vi "LoadRecalcSave.vi"(6 "Segments":bool[](array[boolean]), 8 "Time":string, 9 "Segments(s)":dbl[](array[numeric]), 10 "LoadBackPath":path, 11 "Slide in":refnum<vi>) -> (2 "ForAnalysisPath":path, 3 "ForSegmentsBMP":path)   [LabVIEW 2018]
uses:
  <vilib>/Utility/file.llb/Write Delimited Spreadsheet (string).vi
  Globaltracker.vi
panel:
  out "TTLIsActive":bool
  out "TTLOn":i32
  out "Counter":i32
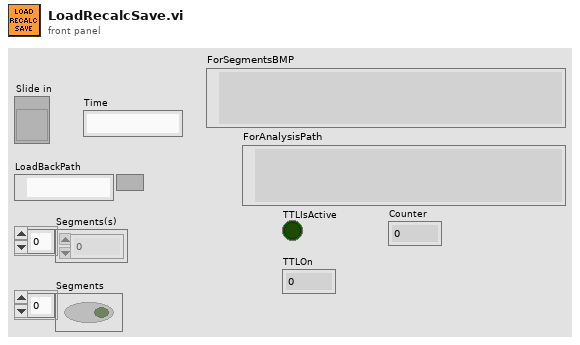
[diagram p1: front panel]
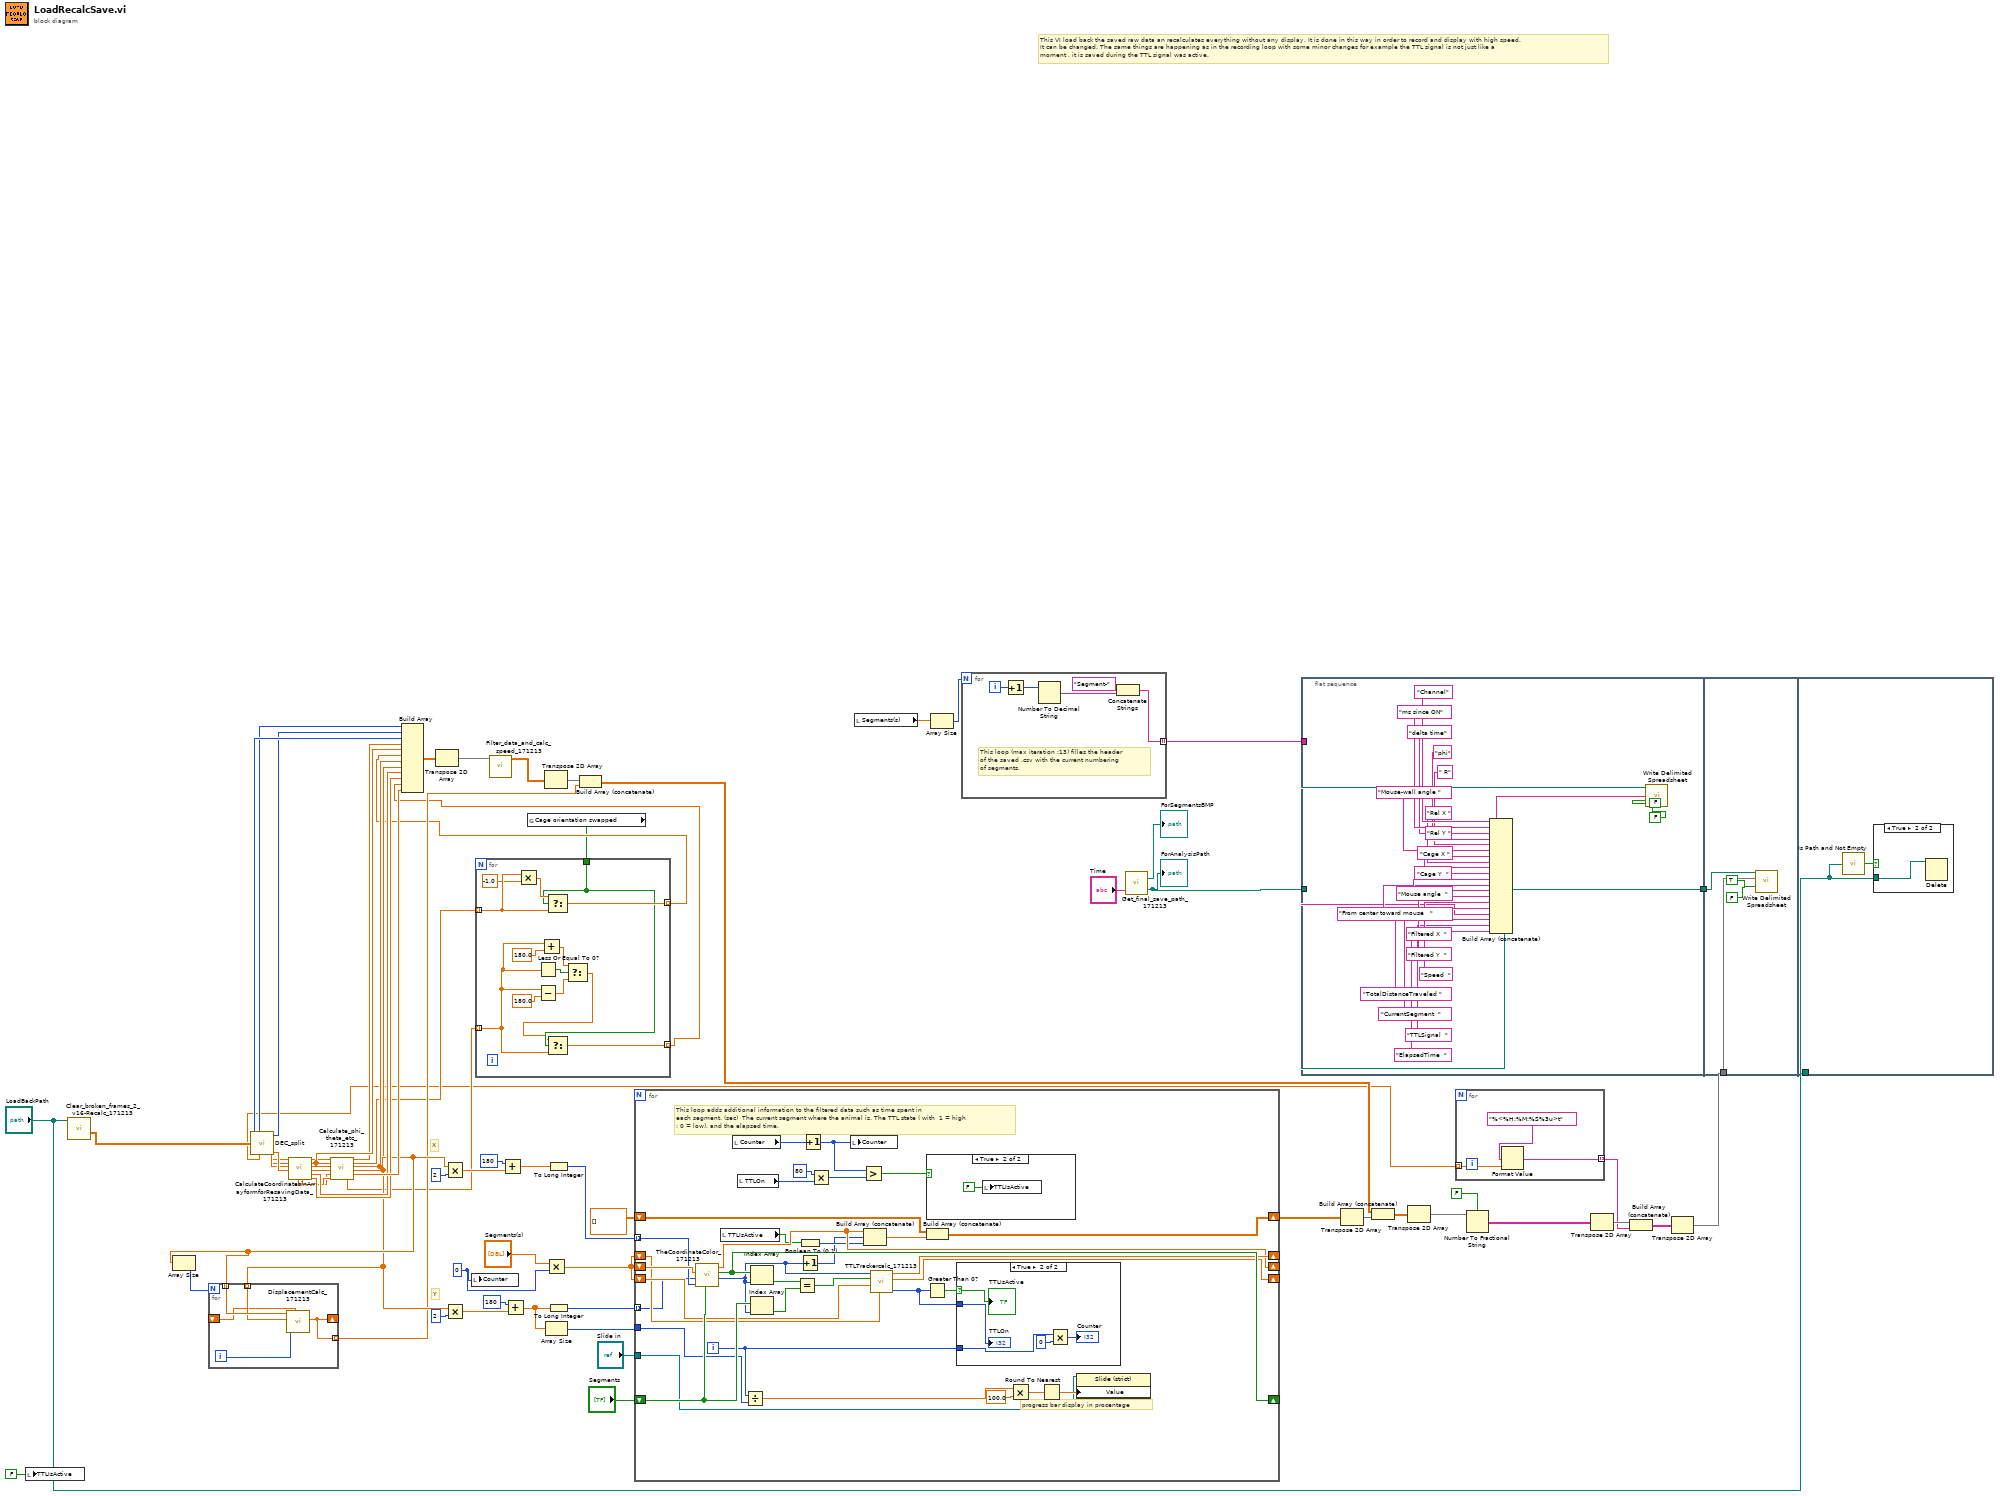
[diagram p0: block diagram]
diagram:
  w23 = 0 ("index")
  # "This VI load back the saved raw data an recalculates everything without any display. It is done in this way in order to record and display with high speed. \nIt can be changed. The same things are happening as in the recording loop with some minor changes for example the TTL signal is not just like a\nmoment , it is saved during the TTL signal was active."
  # "Y"
  # "X"
  n1 = local write "TTLIsActive"(FALSE ("TTLIsActive")) -> ()
  n2 = call "Clear_broken_frames_2_v16-Recalc_171213.vi"("file path (dialog if empty)"="LoadBackPath") -> ("Cleaned array"=w16:dbl[][])  [unwired: 8 in, 2 out]
  n3 = call "DEC_split.vi"("Input DEC array"=w16) -> ("ms since ON"=w39:u32[], "Channel"=w38:u32[], "delta time"=w40:u32[], "Timepoint"=w1:dbl[], "X1"=w29:sgl[], "Y1"=w30:sgl[], "X2"=w31:sgl[], "Y2"=w32:sgl[])  [unwired: 2 out]
  n4 = call "CalculateCoordinatesinArrayformforResavingData_171213.vi"("X1"=w29, "Y1"=w30, "X2"=w31, "Y2"=w32) -> ("X1-X2"=w36:sgl[], "Y1-Y2"=w37:sgl[], "sin(a)"=w33:sgl[], "R from center"=w42:sgl[], "Mouse Xc"=w34:sgl[], "Mouse Yc"=w35:sgl[], "Cage Xc"=w43:sgl[], "Cage Yc"=w44:sgl[])  [unwired: 8 in]
  n5 = call "Calculate_phi_theta_etc_171213.vi"("sin(a)"=w33, "R from center"=w42, "Mouse Xc"=w34, "Mouse Yc"=w35, "X1-X2"=w36, "Y1-Y2"=w37) -> ("Mouse-angle"=w7:dbl[], "phi"=w41:dbl[], "Mouse-wall angle"=w6:dbl[], "Rel X"=w13:dbl[], "Rel Y"=w12:dbl[], "From center towards mouse"=w45:dbl[])  [unwired: 7 in, 1 out]
  n6 = Array Size(array=w13) -> (size(s)=w14:i32)
  n7 = for {
    N: w14 -> [_]
    tunnel: w13 -> [w73] mode=indexing
    tunnel: w12 -> [w72] mode=indexing
    shift-right: [w70] -> _
    shift-left: _ -> [w71]
    tunnel: [w70] -> w9 mode=indexing
    i -> [w74]
    n8 = call "DisplacementCalc_171213.vi"("TotalDistanceTraveledInput"=w71, "i"=w74, "Y"=w72, "X"=w73) -> ("TotalDistanceTraveledOutput"=w70:dbl)  [unwired: 6 in, 1 out]
  }
  n9 = Multiply(x=w13, y=2 ("disabled index (col)")) -> (x*y=w49:dbl[])
  n10 = Multiply(x=w12, y=2 ("disabled index (col)")) -> (x*y=w50:dbl[])
  n11 = local write "Counter"(w23) -> ()
  n12 = Add(x=180 ("disabled index (col)"), y=w49) -> (x+y=w53:dbl[])
  n13 = Add(x=180 ("disabled index (col)"), y=w50) -> (x+y=w68:dbl[])
  n14 = global read "Globaltracker.vi" "Cage orientation swapped"() -> (w4:bool)
  n15 = for {
    tunnel: w7 -> [w76] mode=indexing
    tunnel: w6 -> [w85] mode=indexing
    tunnel: [w87] -> w5 mode=indexing
    tunnel: w4 -> [w82]
    tunnel: [w83] -> w3 mode=indexing
    n16 = Multiply(x=w85, y=-1.0) -> (x*y=w86:dbl)
    n17 = Less Or Equal To 0?(x=w76) -> (x <= 0?=w81:bool)
    n18 = Subtract(x=w76, y=180.0) -> (x-y=w77:dbl)
    n19 = Add(x=w76, y=180.0) -> (x+y=w80:dbl)
    n20 = Select(t=w86, s=w82, f=w85) -> (s? t:f=w87:dbl)
    n21 = Select(t=w80, s=w81, f=w77) -> (s? t:f=w79:dbl)
    n22 = Select(t=w79, s=w82, f=w76) -> (s? t:f=w83:dbl)
  }
  n23 = Build Array ("Pack to array")(w38, w39, w40, w41, w42, w5, w13, w12, w43, w44, w3, w45) -> (w46:dbl[][])
  n24 = Transpose 2D Array(2D array=w46) -> (transposed array=w67:dbl[][])
  n25 = call "Filter_data_and_calc_speed_171213.vi"("Input array (clean)"=w67) -> ("Output"=w11:dbl[][])  [unwired: 10 in]
  n26 = Transpose 2D Array(2D array=w11) -> (transposed array=w10:dbl[][])
  n27 = Multiply(x="Segments(s)", y=w23) -> (x*y=w56:dbl[])
  n28 = Array Size(array=w68) -> (size(s)=w69:i32)
  n29 = To Long Integer(number=w53) -> (32bit integer=w54:i32[])
  n30 = To Long Integer(number=w68) -> (32bit integer=w65:i32[])
  n31 = Build Array (concatenate)(w10, w9) -> (w8:dbl[][])
  n32 = for {
    tunnel: w54 -> [w90] mode=indexing
    tunnel: w65 -> [w89] mode=indexing
    shift-right: [w112] -> _
    shift-left: w56 -> [w122]
    shift-right: [w115] -> _
    shift-left: w56 -> [w116]
    shift-right: [w113] -> _
    shift-left: w56 -> [w114]
    shift-right: [w118] -> _
    shift-left: "Segments" -> [w119]
    shift-right: [w109] -> w63
    shift-left: dbl[][] [] -> [w108]
    tunnel: w69 -> [w91]
    tunnel: "Slide in" -> [w101]
    i -> [w88]
    # "This loop adds additional information to the filtered data such as time spent in \neach segment. (sec)  The current segment where the animal is. The TTL state ( with  1 = high\n; 0 = low), and the elapsed time."
    # "progress bar display in procentage"
    n33 = call "TheCoordinateColor_171213.vi"("InputSegments"=w119, "X"=w90, "Y"=w89, "InputSegments(s)"=w122) -> ("MATCH index"=w111:i32, "Outputsegments"=w118:bool[], "OutputSegmens(s)"=w112:dbl[])  [unwired: 5 in]
    n34 = local read "TTLIsActive"() -> (w92:bool)
    n35 = local read "Counter"() -> (w99:i32)
    n36 = local read "TTLOn"() -> (w96:i32)
    n37 = Divide(x=w88, y=w91) -> (x/y=w103:dbl)
    n38 = Index Array(array=w118, index=w111) -> (element=w120:bool)
    n39 = Index Array(array=w119, index=w111) -> (element=w121:bool)
    n40 = Equal?(x=w120, y=w121) -> (x = y?=w117:bool)
    n41 = Boolean To (0,1)(Boolean=w92) -> (0, 1=w110:i16)
    n42 = Increment(x=w111) -> (x+1=w106:i32)
    n43 = Increment(x=w99) -> (x+1=w93:i32)
    n44 = Multiply(x=80, y=w96) -> (x*y=w94:i32)
    n45 = local write "Counter"(w93) -> ()
    n46 = Greater?(x=w93, y=w94) -> (0:w98:bool)
    n47 = Build Array (concatenate)(w112, w106, w110) -> (w107:dbl[])
    n48 = call "TTLTrackercalc_171213.vi"("Outside in"=w114, "Inside in"=w116, "Boolean"=w117, "MATCH index"=w111) -> ("TTLduration"=w97:i32, "Inside out"=w115:dbl[], "Outside out"=w113:dbl[])  [unwired: 5 in]
    n49 = Greater Than 0?(x=w97) -> (x > 0?=w100:bool)
    n50 = case shown="True" w98 {
      frame False {
      }
      frame True {
        n51 = local write "TTLIsActive"(FALSE ("RewardanalyzeON")) -> ()
      }
    }
    n52 = Build Array (concatenate)(w108, w107) -> (w109:dbl[][])
    n53 = case shown="True" w100 {
      selector: w100 -> [_ w124]
      tunnel: w88 -> [_ w128]
      tunnel: w97 -> [_ w125]
      frame False {
      }
      frame True {
        n54 = Multiply(x=w128, y=0) -> (x*y=→"Counter":i32)
        "TTLOn" <- w125
        "TTLIsActive" <- w124
      }
    }
    n55 = Multiply(x=w103, y=100.0) -> (x*y=w105:dbl)
    n56 = Round To Nearest(number=w105) -> (nearest integer value=w102:dbl)
    n57 = property class="Slide (strict)"(reference=w101, "Value"=w102) -> ()  [unwired: 1 in, 2 out]
  }
  n58 = local read "Segments(s)"() -> (w21:dbl[])
  n59 = Array Size(array=w21) -> (size(s)=w20:i32)
  n60 = for {
    N: w20 -> [_]
    tunnel: [w130] -> w19 mode=indexing
    i -> [w132]
    # "This loop (max iteration :13) filles the header\nof the saved .csv with the current numbering\nof segments."
    n61 = Increment(x=w132) -> (x+1=w129:i32)
    n62 = Number To Decimal String(number=w129) -> (decimal integer string=w131:string)  [unwired: 1 in]
    n63 = Concatenate Strings("Segment-", w131) -> (w130:string)
  }
  n64 = call "Get_final_save_path_171213.vi"("Time string"="Time") -> ("File output path"=w24:path, "For regions"=→"ForSegmentsBMP":path)  [unwired: 2 in]
  "ForAnalysisPath" <- w24
  n65 = flat-sequence {
    tunnel: w24 -> [w155]
    tunnel: [w155] -> w27
    tunnel: w19 -> [w137]
    tunnel: w27 -> [w161]
    tunnel: w22 -> [w160]
    tunnel: "LoadBackPath" -> [w163]
    frame #0 {
      n66 = Build Array (concatenate)("Channel", "ms since ON", "delta time", "phi", " R", "Mouse-wall angle ", "Rel X ", "Rel Y ", "Cage X ", "Cage Y  ", "Mouse angle  ", "From center toward mouse   ", "Filtered X  ", "Filtered Y  ", "Speed  ", "TotalDistanceTraveled ", w137, "CurrentSegment  ", "TTLSignal  ", "ElapsedTime  ") -> (w138:string[])
      n67 = call-poly <vilib>:"Write Delimited Spreadsheet.vi"("file path (dialog if empty)"=w155, "1D data"=w138, "append to file? (new file:F)"=FALSE, "transpose? (no:F)"=FALSE) -> ()  [unwired: 10 in, 2 out]
    }
    frame #1 {
      n68 = call-poly <vilib>:"Write Delimited Spreadsheet.vi"("file path (dialog if empty)"=w161, "2D data"=w160, "append to file? (new file:F)"=TRUE, "transpose? (no:F)"=FALSE ("append to file? (new file:F)")) -> ()  [unwired: 10 in, 2 out]
    }
    frame #2 {
      n69 = call <vilib>:"Is Path and Not Empty.vi"("path"=w163) -> ("Is Path and Not Empty?"=w162:bool)  [unwired: 4 in]
      n70 = case shown="True" w162 {
        tunnel: w163 -> [_ w164]
        frame False {
        }
        frame True {
          n71 = Delete(path (use dialog)=w164) -> ()  [unwired: 4 in, 3 out]
        }
      }
    }
  }
  n72 = Transpose 2D Array(2D array=w63) -> (transposed array=w58:dbl[][])
  n73 = Build Array (concatenate)(w8, w58) -> (w59:dbl[][])
  n74 = Transpose 2D Array(2D array=w59) -> (transposed array=w64:dbl[][])
  n75 = for {
    tunnel: w1 -> [w167] mode=indexing
    tunnel: [w166] -> w2 mode=indexing
    n76 = Format Value(format string="%<%H:%M:%S%3u>t", value (0)=w167) -> (output string=w166:string)  [unwired: 1 in]
  }
  n77 = Number To Fractional String(use system decimal point (T)=FALSE, number=w64) -> (F-format string=w62:string[][])  [unwired: 2 in]
  n78 = Transpose 2D Array(2D array=w62) -> (transposed array=w61:string[][])
  n79 = Build Array (concatenate)(w61, w2) -> (w60:string[][])
  n80 = Transpose 2D Array(2D array=w60) -> (transposed array=w22:string[][])
